vi "Index_Write.vi"(8 "error in (no error)":errorcluster, 11 "Index":T1) -> (0 "error out":errorcluster)   [LabVIEW 2016, in "SeqProcessor.lvlib"]
uses:
  SeqProcessor.lvlib
  controls/StepIndex.ctl
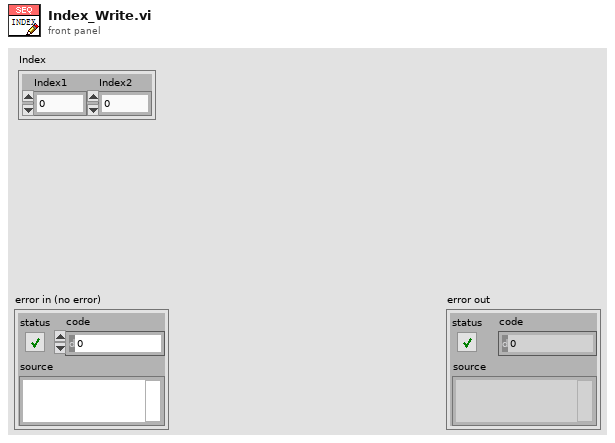
[diagram p1: front panel]
types:
  T1 = typedef "SeqProcessor.lvlib/StepIndex.ctl" = cluster{"Index1":u32, "Index2":u32}
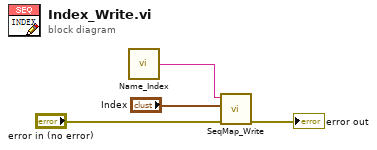
[diagram p0: block diagram]
diagram:
  n1 = call "Name_Index.vi"() -> ("StepIndex"=w2:string)  [unwired: 5 in]
  n2 = call "SeqMap_Write.vi"("error in (no error)"="error in (no error)", "Value"="Index", "Tag"=w2) -> ("error out"=→"error out":errorcluster)  [unwired: 8 in]
